vi "checkTimeOut.vi"(8 "error in (no error)":errorcluster, 10 "Time":u32, 11 "ParameterConf in":refnum<class "ParameterConf.lvclass">) -> (0 "error out":errorcluster, 1 "stateDisplay":T1, 2 "timeout":bool, 3 "ParameterConf out":refnum<class "ParameterConf.lvclass">)   [LabVIEW 2014, in "LibraryGcode.lvlib" / "ParameterConf.lvclass"]
uses:
  ParameterConf.lvclass
  stateLoop_View.ctl
  ParameterConf.lvclass/ParameterConf.ctl
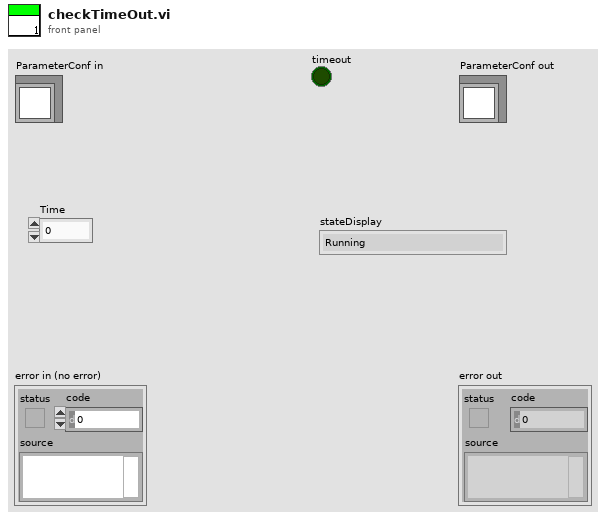
[diagram p1: front panel]
types:
  T1 = typedef "LibraryGcode.lvlib/ParameterConf.lvclass/stateLoop_View.ctl" = enum16{"Running", "writeGlobal", "schedules500ms", "init", "End"}
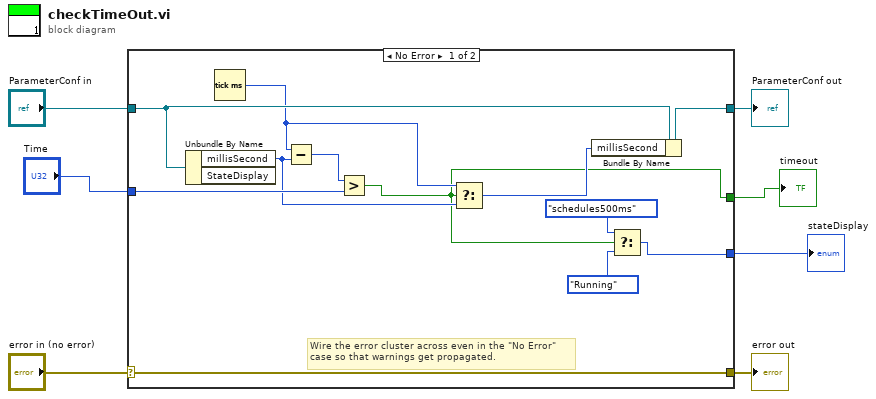
[diagram p0: block diagram]
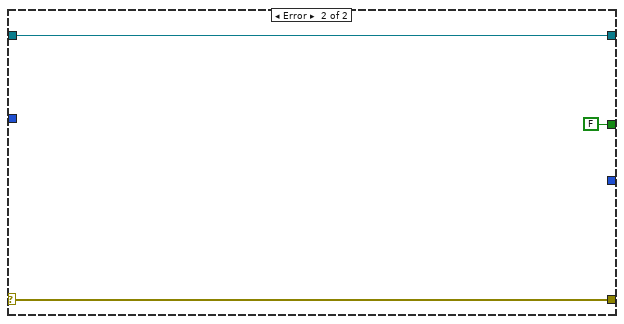
[diagram p2: hidden frame]
diagram:
  n1 = case shown="No Error" "error in (no error)" {
    selector: "error in (no error)" -> [w19 w22]
    tunnel: [w19 w22] -> w6
    tunnel: [w16 w21] -> w4
    tunnel: "ParameterConf in" -> [w17 w21]
    tunnel: "Time" -> [w13 _]
    tunnel: [w9 FALSE] -> w2
    tunnel: [w8 _] -> w1
    frame No Error {
      # "Wire the error cluster across even in the \"No Error\"\ncase so that warnings get propagated."
      n2 = Unbundle By Name(w17) -> ("millisSecond"=w12:u32)  [unwired: 1 out]
      n3 = Tick Count (ms)() -> (millisecond timer value=w14:u32)
      n4 = Subtract(x=w14, y=w12) -> (x-y=w18:u32)
      n5 = Greater?(x=w18, y=w13) -> (0:w9:bool)
      n6 = Select(t=w14, s=w9, f=w12) -> (s? t:f=w15:u32)
      n7 = Bundle By Name(cluster=w17, "millisSecond"=w15) -> (w16:refnum<class "ParameterConf.lvclass">)
      n8 = Select(t=stateLoop_View."schedules500ms" ("StateDisplay"), s=w9, f=stateLoop_View."Running" ("StateDisplay")) -> (s? t:f=w8:T1)
    }
    frame Error {
    }
  }
  "error out" <- w6
  "ParameterConf out" <- w4
  "timeout" <- w2
  "stateDisplay" <- w1
